vi "Coerce Stimulus Interval.vi"(8 "error in (no error)":errorcluster, 9 "AI sampling rate (Hz)":dbl format="%#_10g", 10 "AO sampling rate (Hz)":dbl format="%#_10g", 11 "Stimulus interval (ms)":dbl) -> (0 "error out":errorcluster, 1 "AI npts":i32, 2 "AO npts":i32, 3 "Coerced interval (ms)":dbl)   [LabVIEW 2020]
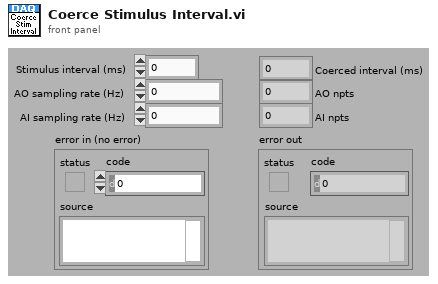
[diagram p1: front panel]
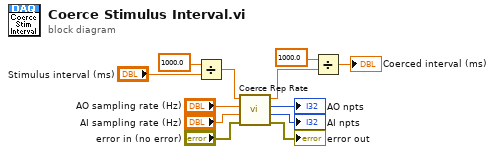
[diagram p0: block diagram]
diagram:
  n1 = Divide(x=1000.0, y="Stimulus interval (ms)") -> (x/y=w10:dbl)
  n2 = call "Coerce Rep Rate.vi"("error in (no error)"="error in (no error)", "AI sampling rate (Hz)"="AI sampling rate (Hz)", "AO sampling rate (Hz)"="AO sampling rate (Hz)", "Rep rate (Hz)"=w10) -> ("error out"=→"error out":errorcluster, "AI npts"=→"AI npts":i32, "AO npts"=→"AO npts":i32, "Coerced rep rate (Hz)"=w3:dbl)  [unwired: 4 in]
  n3 = Divide(x=1000.0, y=w3) -> (x/y=→"Coerced interval (ms)":dbl)
